vi "pulse_generator_refnum_2.vi"(1 "Stop! Refnum":refnum<vi>) -> ()   [LabVIEW 2017]
uses:
  pulse_generator_controls_refnums.ctl
  <vilib>/Utility/error.llb/DialogType.ctl
  <vilib>/DAQmx/write.llb/DAQmx Write (Digital Bool 1Line 1Point).vi
  <vilib>/DAQmx/create/channels.llb/DAQmx Create Channel (DO-Digital Output).vi
  <vilib>/DAQmx/miscellaneous.llb/DAQmx Fill In Error Info.vi
  <vilib>/DAQmx/create/channels.llb/DAQmx Create Channel (CO-Pulse Generation-Frequency).vi
  <vilib>/DAQmx/configure/timing.llb/DAQmx Timing (Implicit).vi
panel:
  in  "Pulse Generator Control Refnums":T1
  out "Stopped!":bool caption="OK"
  in  "Stop! Local":bool
  out "message":string=" INSTRUCTIONS:\r\rNormal Use:  When using subVIs that incorporate the error in/error out (or error I/O) structure, place this handler where you want to inform the user of an error, typically at the end of the I/O data path, as the last action of the program.  If the error in error? is ERROR, the handler creates a message describing the error and its source.  If the type of dialog = 1 (default), the message is displayed to the user, who can only acknowedge it.  If the type = 2, the user can acknowledge the message or abort execution; aborting a program with active I/O is not recommended.  If the type = 0, no message is displayed; this is used to process the error programmatically, and the error out cluster elements are wired to individual terminals for that reason.  \r\rOther Use:\n\r\nlocal testing.  To test the error code of a subVI or function that does not have the error I/O structure, you can wire its error code and a source string to the local error code and error source inputs.  If error in error? indicates no error and error code is not equal to 0, the local code and source are substituted for the error in values, and error? is set TRUE (ERROR)."
  in  "SwitchHelper":bool
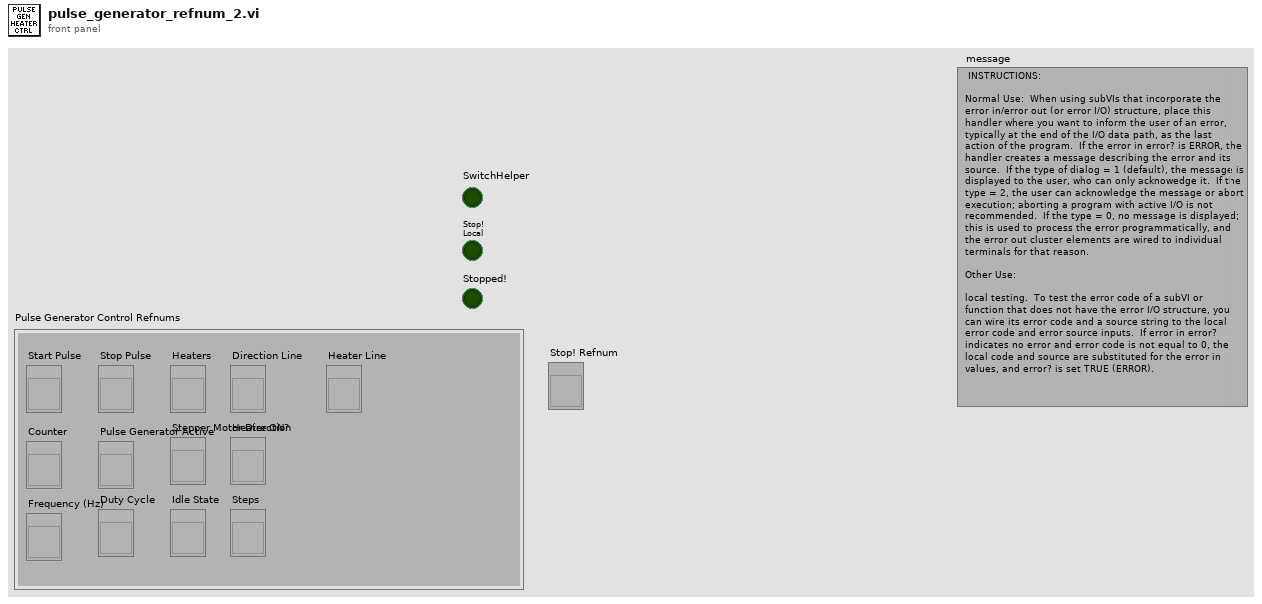
[diagram p1: front panel]
types:
  T1 = typedef "pulse_generator_controls_refnums.ctl" = cluster{"Start Pulse":refnum<vi>, "Stop Pulse":refnum<vi>, "Heaters":refnum<vi>, "Counter":refnum<vi>, "Frequency (Hz)":refnum<vi>, "Duty Cycle":refnum<vi>, "Idle State":refnum<vi>, "Pulse Generator Active":refnum<vi>, "Stepper Motor Direction":refnum<vi>, "Steps":refnum<vi>, "Direction Line":refnum<vi>, "Heater Line":refnum<vi>, "Heater ON?":refnum<vi>}
  T2 = enum8{"Enabled", "Disabled", "Disabled and Grayed Out"}
  T3 = typedef "DialogType.ctl" = u16
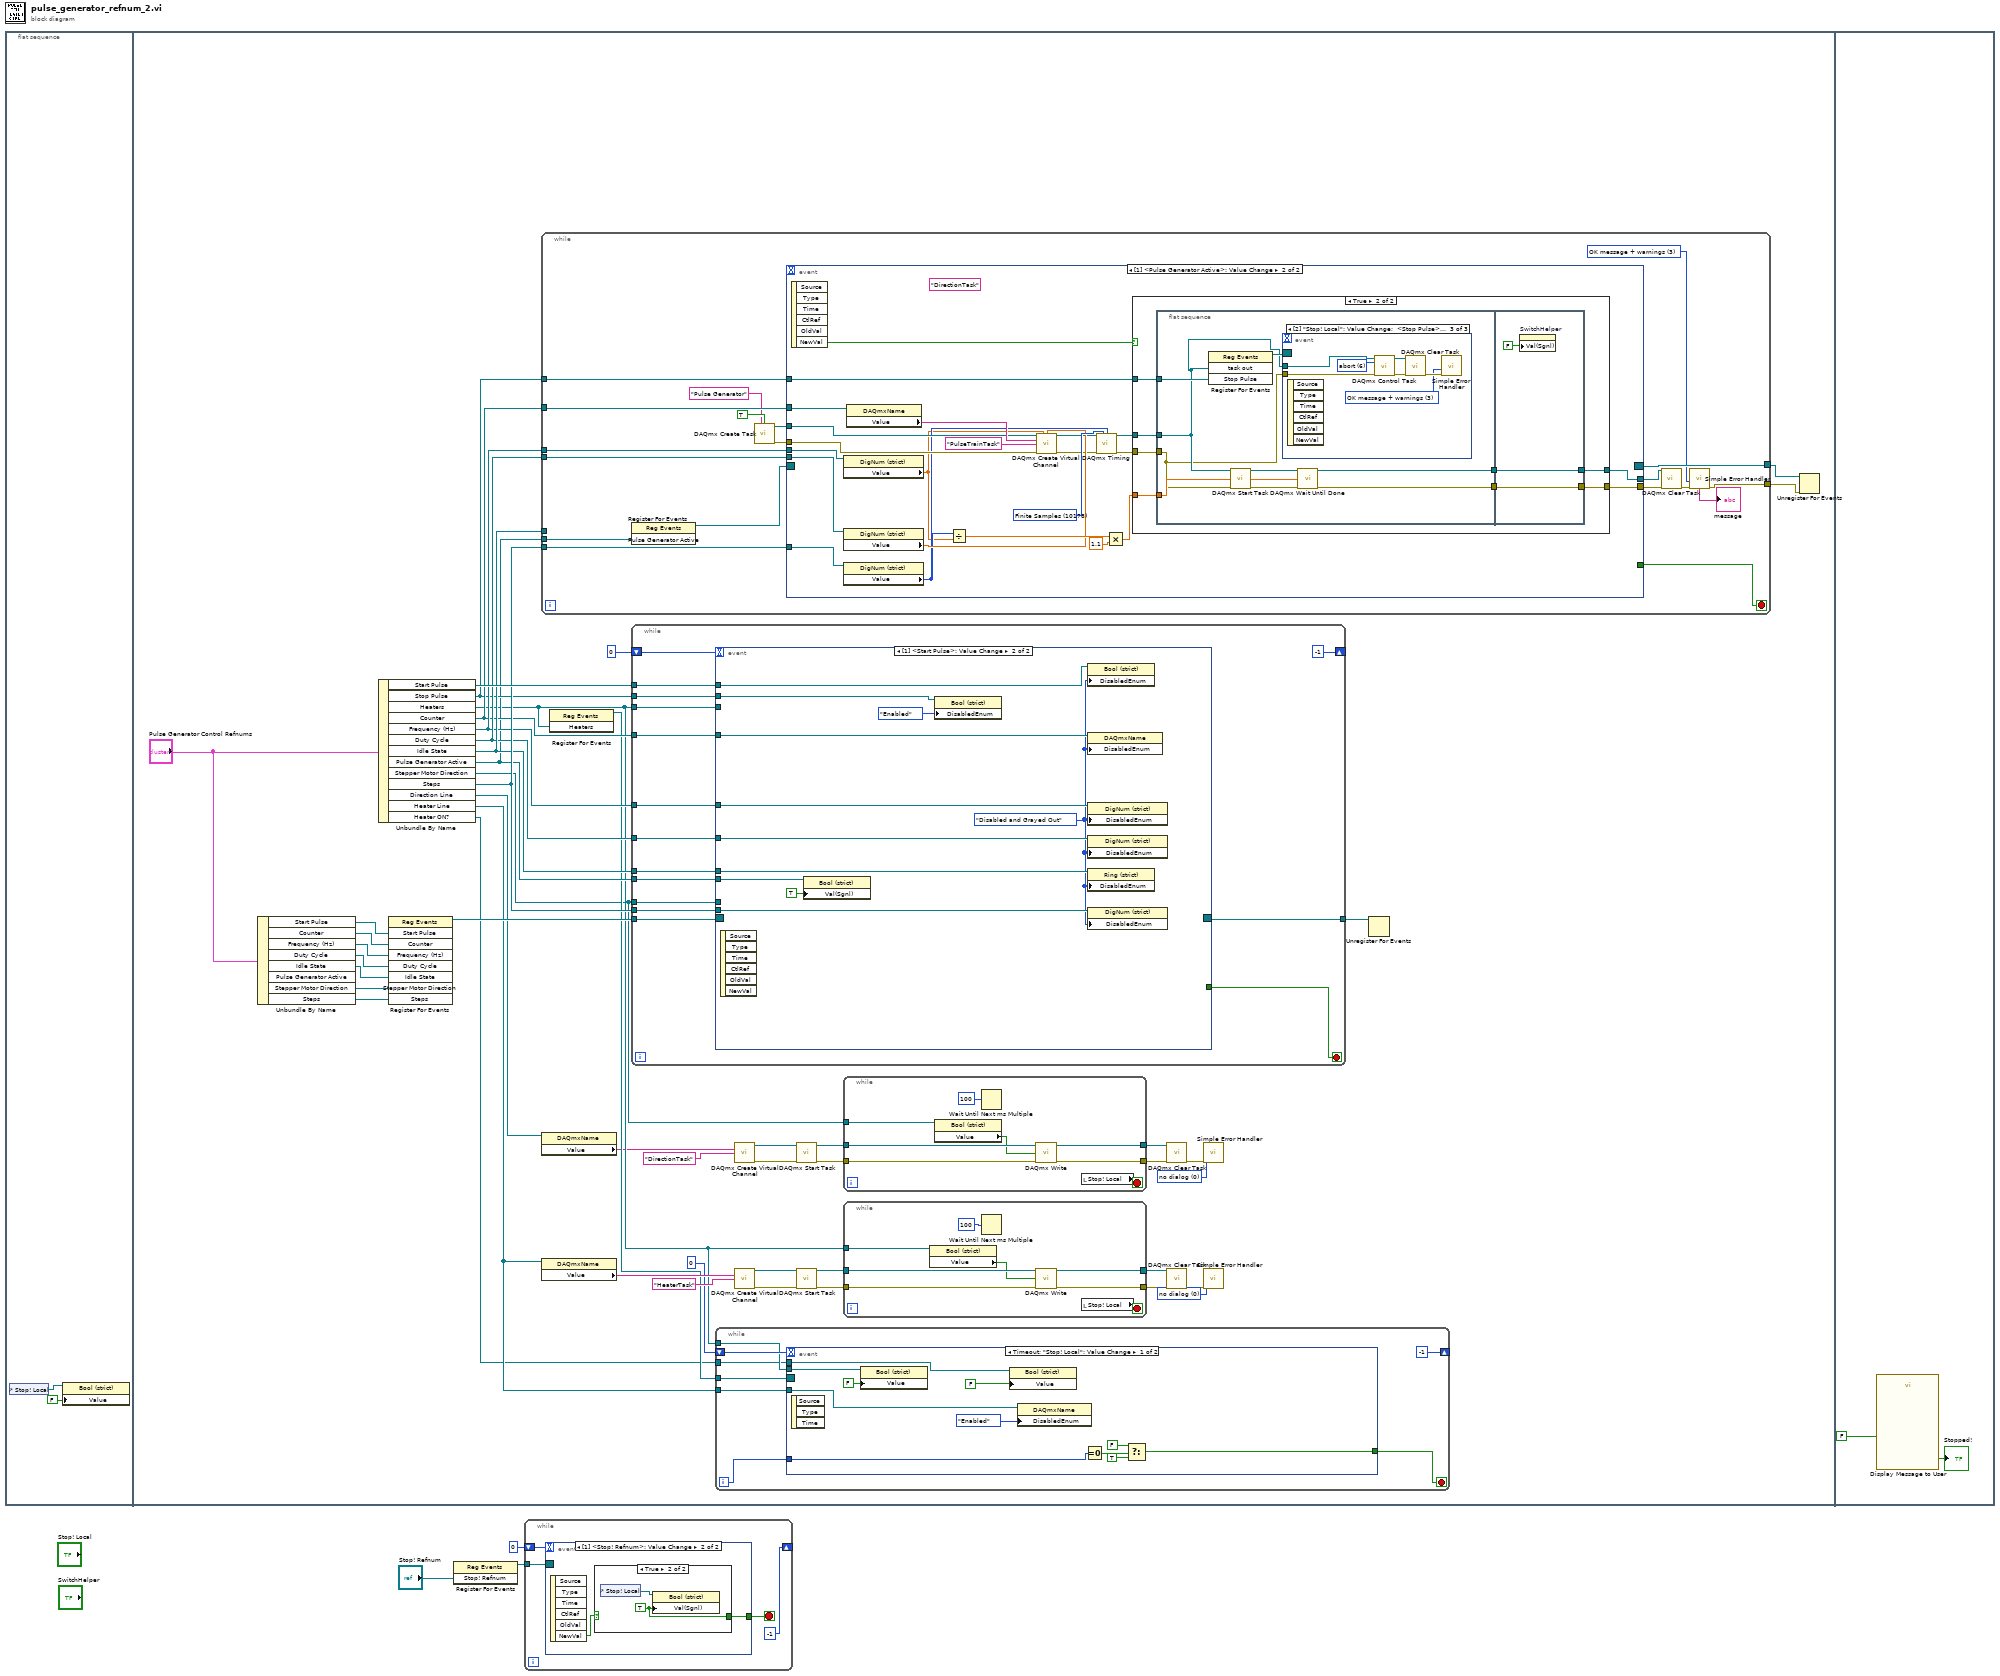
[diagram p0: block diagram]
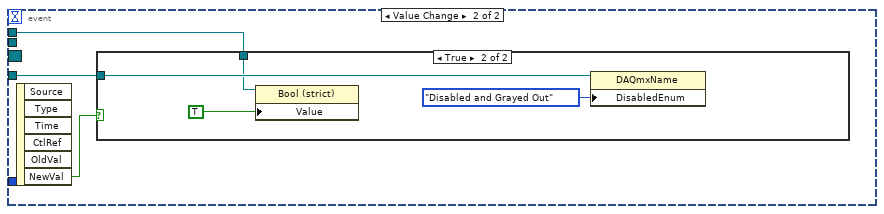
[diagram p2: hidden frame]
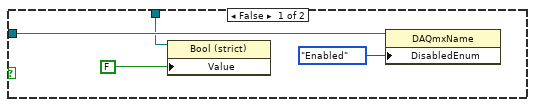
[diagram p3: hidden frame]
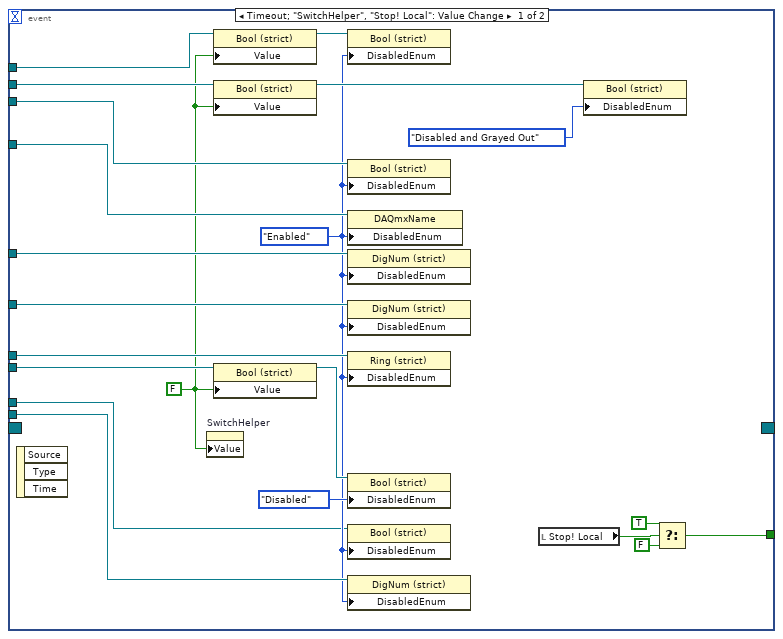
[diagram p4: hidden frame]
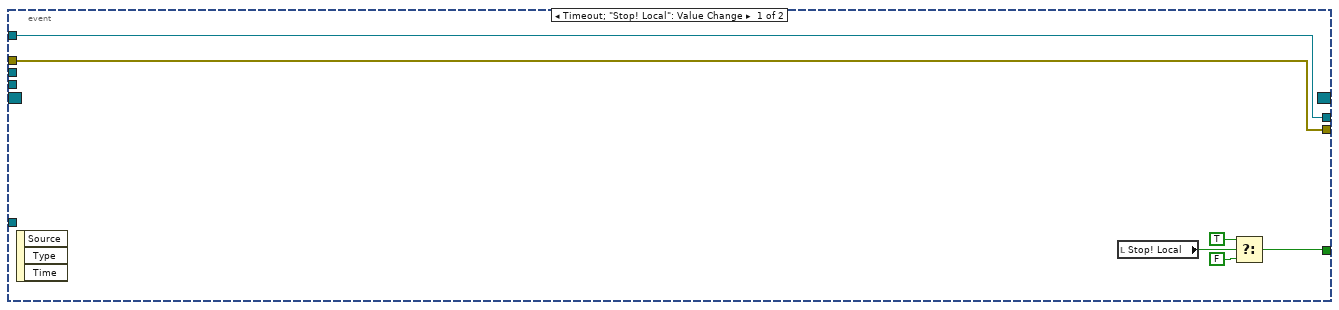
[diagram p5: hidden frame]
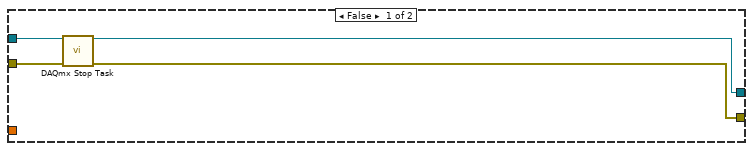
[diagram p6: hidden frame]
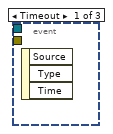
[diagram p7: hidden frame]
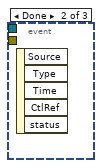
[diagram p8: hidden frame]
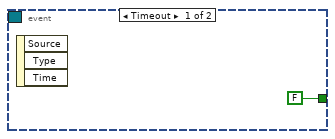
[diagram p9: hidden frame]
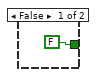
[diagram p10: hidden frame]
diagram:
  n1 = flat-sequence {
    frame #0 {
      n2 = control-ref of="Stop! Local"() -> (w4:refnum<vi>)
      n3 = property class="Bool (strict)"(reference=w4, "Value"=FALSE) -> ()  [unwired: 1 in, 2 out]
    }
    frame #1 {
      w9 = T3 0 items=["no dialog", "OK message", "continue or stop message", "OK message + warnings", "continue/stop + warnings"] ("type of dialog (OK msg:1)")
      w10 = T3 0 items=["no dialog", "OK message", "continue or stop message", "OK message + warnings", "continue/stop + warnings"] ("type of dialog (OK msg:1)")
      n4 = Unbundle By Name("Pulse Generator Control Refnums") -> ("Start Pulse"=w36:refnum<vi>, "Counter"=w51:refnum<vi>, "Frequency (Hz)"=w50:refnum<vi>, "Duty Cycle"=w49:refnum<vi>, "Idle State"=w48:refnum<vi>, "Stepper Motor Direction"=w45:refnum<vi>, "Steps"=w44:refnum<vi>)  [unwired: 1 out]
      n5 = Unbundle By Name("Pulse Generator Control Refnums") -> ("Start Pulse"=w52:refnum<vi>, "Stop Pulse"=w38:refnum<vi>, "Heaters"=w23:refnum<vi>, "Counter"=w39:refnum<vi>, "Frequency (Hz)"=w40:refnum<vi>, "Duty Cycle"=w41:refnum<vi>, "Idle State"=w42:refnum<vi>, "Pulse Generator Active"=w37:refnum<vi>, "Stepper Motor Direction"=w12:refnum<vi>, "Steps"=w43:refnum<vi>, "Direction Line"=w13:refnum<vi>, "Heater Line"=w25:refnum<vi>, "Heater ON?"=w8:refnum<vi>)
      n6 = register-events(w36, w51, w50, w49, w48, w45, w44) -> (reference out=w47:refnum<event-registration>)  [unwired: 2 in, 1 out]
      n7 = while {
        tunnel: w37 -> [w160]
        tunnel: [w162] -> w11
        tunnel: w43 -> [w155]
        tunnel: w42 -> [_]
        tunnel: w41 -> [w153]
        tunnel: w40 -> [w150]
        tunnel: w39 -> [w154]
        tunnel: w38 -> [w161]
        tunnel: [w148] -> w7
        stop <- w149 stop-if-true
        w157 = T3 3 items=["no dialog", "OK message", "continue or stop message", "OK message + warnings", "continue/stop + warnings"] ("type of dialog (OK msg:1)")
        n8 = register-events(w160) -> (reference out=w159:refnum<event-registration>)  [unwired: 2 in, 1 out]
        n9 = call <vilib>:"DAQmx Create Task.vi"("new task name"="Pulse Generator", "auto cleanup"=TRUE) -> ("task out"=w152:refnum<k21>, "error out"=w151:errorcluster)  [unwired: 12 in]
        n10 = event shown="[1] <Pulse Generator Active>: Value Change" {
          selector: w159 -> [_ _]
          dyn-events: [_ _] -> w162
          timeout: _ -> [_ _]
          tunnel: [w170 w192] -> w164
          tunnel: [w171 w193] -> w163
          tunnel: w152 -> [w171 w179]
          tunnel: w151 -> [w170 w178]
          tunnel: w161 -> [_ w191]
          tunnel: w155 -> [_ w184]
          tunnel: w154 -> [_ w182]
          tunnel: w153 -> [_ w180]
          tunnel: w150 -> [_ w172]
          tunnel: [w166 _] -> w149
          event Timeout; "Stop! Local": Value Change {
            n11 = event-data() -> ()  [unwired: 1 in, 3 out]
            n12 = local read "Stop! Local"() -> (w167:bool)
            n13 = Select(t=TRUE ("Value"), s=w167, f=FALSE ("Value")) -> (s? t:f=w166:bool)
          }
          event Value Change {
            (unwired) "DirectionTask" ("name to assign")
            w188 = 10178 items=["Finite Samples"=10178, "Continuous Samples"=10123, "Hardware Timed Single Point"=12522] ("sample mode")
            n14 = event-data() -> ("NewVal"=w194:bool)  [unwired: 1 in, 5 out]
            n15 = property class="DigNum (strict)"(reference=w172) -> ("Value"=w173:dbl)  [unwired: 1 in, 2 out]
            n16 = property class="DigNum (strict)"(reference=w180) -> ("Value"=w181:dbl)  [unwired: 1 in, 2 out]
            n17 = property class="DigNum (strict)"(reference=w184) -> ("Value"=w177:i32)  [unwired: 1 in, 2 out]
            n18 = property class="DAQmxName"(reference=w182) -> ("Value"=w183:string)  [unwired: 1 in, 2 out]
            n19 = Divide(x=w177, y=w173) -> (x/y=w186:dbl)
            n20 = call-poly <vilib>:"DAQmx Create Virtual Channel.vi"("task in"=w179, "frequency"=w173, "duty cycle"=w181, "counter"=w183, "name to assign"="PulseTrainTask", "error in"=w178) -> ("task out"=w175:refnum<k21>, "error out"=w174:errorcluster)  [unwired: 8 in]
            n21 = call-poly <vilib>:"DAQmx Timing.vi"("task/channels in"=w175, "sample mode"=w188, "samples per channel"=w177, "error in"=w174) -> ("task out"=w190:refnum<k21>, "error out"=w189:errorcluster)  [unwired: 10 in]
            n22 = Multiply(x=w186, y=1.1) -> (x*y=w185:dbl)
            n23 = case shown="True" w194 {
              tunnel: w190 -> [w198 w203]
              tunnel: w189 -> [w197 w206]
              tunnel: [w196 w205] -> w193
              tunnel: [w195 w204] -> w192
              tunnel: w191 -> [_ w200]
              tunnel: w185 -> [_ w199]
              frame False {
                n24 = call <vilib>:"DAQmx Stop Task.vi"("task/channels in"=w198, "error in"=w197) -> ("task out"=w196:refnum<k21>, "error out"=w195:errorcluster)  [unwired: 12 in]
              }
              frame True {
                n25 = flat-sequence {
                  tunnel: w206 -> [w208]
                  tunnel: w203 -> [w209]
                  tunnel: [w214] -> w202
                  tunnel: [w213] -> w201
                  tunnel: w200 -> [w211]
                  tunnel: w199 -> [w210]
                  tunnel: [w224] -> w204
                  tunnel: [w225] -> w205
                  tunnel: w202 -> [w225]
                  tunnel: w201 -> [w224]
                  frame #0 {
                    n26 = register-events(w209, w211) -> (reference out=w212:refnum<event-registration>)  [unwired: 2 in, 1 out]
                    n27 = call <vilib>:"DAQmx Start Task.vi"("task/channels in"=w209, "error in"=w208) -> ("task out"=w215:refnum<k21>, "error out"=w207:errorcluster)  [unwired: 12 in]
                    n28 = event shown="[2] \"Stop! Local\": Value Change;  <Stop Pulse>: Value Change" {
                      selector: w212 -> [_ _ _]
                      dyn-events: _ -> [_ _ _]
                      timeout: _ -> [_ _ _]
                      tunnel: w209 -> [_ _ w222]
                      tunnel: w208 -> [_ _ w221]
                      event Timeout {
                        n29 = event-data() -> ()  [unwired: 1 in, 3 out]
                      }
                      event Done {
                        n30 = event-data() -> ()  [unwired: 1 in, 5 out]
                      }
                      event "Stop! Local": Value Change {
                        w216 = T3 3 items=["no dialog", "OK message", "continue or stop message", "OK message + warnings", "continue/stop + warnings"] ("type of dialog (OK msg:1)")
                        w220 = 6 items=["verify"=2, "reserve"=4, "commit"=3, "unreserve"=5, "abort"=6] ("action")
                        n31 = event-data() -> ()  [unwired: 1 in, 6 out]
                        n32 = call <vilib>:"DAQmx Control Task.vi"("task/channels in"=w222, "action"=w220, "error in"=w221) -> ("task out"=w219:refnum<k21>, "error out"=w218:errorcluster)  [unwired: 11 in]
                        n33 = call <vilib>:"DAQmx Clear Task.vi"("task in"=w219, "error in"=w218) -> ("error out"=w217:errorcluster)  [unwired: 13 in]
                        n34 = call <vilib>:"Simple Error Handler.vi"("type of dialog (OK msg:1)"=w216, "error in (no error)"=w217) -> ()  [unwired: 3 in, 5 out]
                      }
                    }
                    n35 = call <vilib>:"DAQmx Wait Until Done.vi"("task/channels in"=w215, "timeout (sec)"=w210, "error in"=w207) -> ("task out"=w214:refnum<k21>, "error out"=w213:errorcluster)  [unwired: 11 in]
                  }
                  frame #1 {
                    n36 = property on="SwitchHelper" class="Bool (strict)"("Val(Sgnl)"=FALSE ("Value (Signaling)")) -> ()  [unwired: 2 in, 2 out]
                  }
                }
              }
            }
          }
        }
        n37 = call <vilib>:"DAQmx Clear Task.vi"("task in"=w163, "error in"=w164) -> ("error out"=w165:errorcluster)  [unwired: 13 in]
        n38 = call <vilib>:"Simple Error Handler.vi"("type of dialog (OK msg:1)"=w157, "error in (no error)"=w165) -> ("error out"=w148:errorcluster, "message"=→"message":string)  [unwired: 3 in, 3 out]
      }
      n39 = property class="DAQmxName"(reference=w13) -> ("Value"=w15:string)  [unwired: 1 in, 2 out]
      n40 = property class="DAQmxName"(reference=w25) -> ("Value"=w34:string)  [unwired: 1 in, 2 out]
      n41 = register-events(w23) -> (reference out=w26:refnum<event-registration>)  [unwired: 2 in, 1 out]
      n42 = while {
        shift-right: [-1] -> _
        shift-left: 0 -> [w114]
        tunnel: w52 -> [w112]
        tunnel: w38 -> [w111]
        tunnel: w23 -> [w101]
        tunnel: w39 -> [w107]
        tunnel: w40 -> [w106]
        tunnel: w41 -> [w105]
        tunnel: w42 -> [w104]
        tunnel: w37 -> [w110]
        tunnel: w12 -> [w103]
        tunnel: w47 -> [w109]
        tunnel: [w108] -> w46
        tunnel: w43 -> [w102]
        stop <- w100 stop-if-true
        n43 = event shown="[1] <Start Pulse>: Value Change" {
          selector: w109 -> [_ _]
          dyn-events: [_ _] -> w108
          timeout: w114 -> [_ _]
          tunnel: w112 -> [w135 w146]
          tunnel: w111 -> [w134 w140]
          tunnel: w110 -> [w133 w137]
          tunnel: w107 -> [w122 w145]
          tunnel: w106 -> [w124 w141]
          tunnel: w105 -> [w126 w144]
          tunnel: w104 -> [w127 w143]
          tunnel: w103 -> [w120 _]
          tunnel: w102 -> [w125 w142]
          tunnel: w101 -> [w123 _]
          tunnel: [w117 _] -> w100
          event Timeout; "SwitchHelper", "Stop! Local": Value Change {
            w121 = T2."Enabled" ("Disabled")
            w119 = FALSE ("Value")
            n44 = event-data() -> ()  [unwired: 1 in, 3 out]
            n45 = property on="SwitchHelper" class="Bool (strict)"("Value"=w119) -> ()  [unwired: 2 in, 2 out]
            n46 = property class="Bool (strict)"(reference=w135, "Value"=w119) -> (reference out=w132:refnum<vi>)  [unwired: 1 in, 1 out]
            n47 = property class="Bool (strict)"(reference=w134, "Value"=w119) -> (reference out=w131:refnum<vi>)  [unwired: 1 in, 1 out]
            n48 = property class="Bool (strict)"(reference=w133, "Value"=w119) -> (reference out=w130:refnum<vi>)  [unwired: 1 in, 1 out]
            n49 = property class="Bool (strict)"(reference=w132, "DisabledEnum"=w121) -> ()  [unwired: 1 in, 2 out]
            n50 = property class="Bool (strict)"(reference=w123, "DisabledEnum"=w121) -> ()  [unwired: 1 in, 2 out]
            n51 = property class="DAQmxName"(reference=w122, "DisabledEnum"=w121) -> ()  [unwired: 1 in, 2 out]
            n52 = property class="DigNum (strict)"(reference=w124, "DisabledEnum"=w121) -> ()  [unwired: 1 in, 2 out]
            n53 = property class="DigNum (strict)"(reference=w126, "DisabledEnum"=w121) -> ()  [unwired: 1 in, 2 out]
            n54 = property class="Ring (strict)"(reference=w127, "DisabledEnum"=w121) -> ()  [unwired: 1 in, 2 out]
            n55 = property class="Bool (strict)"(reference=w130, "DisabledEnum"=T2."Disabled" ("Disabled")) -> ()  [unwired: 1 in, 2 out]
            n56 = property class="Bool (strict)"(reference=w120, "DisabledEnum"=w121) -> ()  [unwired: 1 in, 2 out]
            n57 = property class="DigNum (strict)"(reference=w125, "DisabledEnum"=w121) -> ()  [unwired: 1 in, 2 out]
            n58 = local read "Stop! Local"() -> (w118:bool)
            n59 = property class="Bool (strict)"(reference=w131, "DisabledEnum"=T2."Disabled and Grayed Out" ("Disabled")) -> ()  [unwired: 1 in, 2 out]
            n60 = Select(t=TRUE ("Value"), s=w118, f=FALSE ("Value")) -> (s? t:f=w117:bool)
          }
          event Value Change {
            w139 = T2."Disabled and Grayed Out" ("Disabled")
            n61 = event-data() -> ()  [unwired: 1 in, 6 out]
            n62 = property class="Bool (strict)"(reference=w137, "Val(Sgnl)"=TRUE ("Value")) -> ()  [unwired: 1 in, 2 out]
            n63 = property class="Bool (strict)"(reference=w140, "DisabledEnum"=T2."Enabled" ("Disabled")) -> ()  [unwired: 1 in, 2 out]
            n64 = property class="Bool (strict)"(reference=w146, "DisabledEnum"=w139) -> ()  [unwired: 1 in, 2 out]
            n65 = property class="DAQmxName"(reference=w145, "DisabledEnum"=w139) -> ()  [unwired: 1 in, 2 out]
            n66 = property class="DigNum (strict)"(reference=w141, "DisabledEnum"=w139) -> ()  [unwired: 1 in, 2 out]
            n67 = property class="DigNum (strict)"(reference=w144, "DisabledEnum"=w139) -> ()  [unwired: 1 in, 2 out]
            n68 = property class="Ring (strict)"(reference=w143, "DisabledEnum"=w139) -> ()  [unwired: 1 in, 2 out]
            n69 = property class="DigNum (strict)"(reference=w142, "DisabledEnum"=w139) -> ()  [unwired: 1 in, 2 out]
          }
        }
      }
      n70 = while {
        tunnel: w26 -> [w69]
        tunnel: w25 -> [w68]
        shift-right: [-1 ("millisecond multiple")] -> _
        shift-left: 0 ("millisecond multiple") -> [w67]
        tunnel: w23 -> [w65]
        tunnel: w8 -> [w62]
        i -> [w64]
        stop <- w63 stop-if-true
        n71 = event shown="[0] Timeout;  \"Stop! Local\": Value Change" {
          selector: w69 -> [_ _]
          dyn-events: _ -> [_ _]
          timeout: w67 -> [_ _]
          tunnel: w68 -> [w79 w82]
          tunnel: w65 -> [w78 _]
          tunnel: w64 -> [w75 _]
          tunnel: [w72 _] -> w63
          tunnel: w62 -> [w70 w81]
          event Timeout; "Stop! Local": Value Change {
            n72 = event-data() -> ()  [unwired: 1 in, 3 out]
            n73 = property class="Bool (strict)"(reference=w78, "Value"=FALSE) -> ()  [unwired: 1 in, 2 out]
            n74 = property class="Bool (strict)"(reference=w70, "Value"=FALSE) -> ()  [unwired: 1 in, 2 out]
            n75 = property class="DAQmxName"(reference=w79, "DisabledEnum"=T2."Enabled" ("Disabled")) -> ()  [unwired: 1 in, 2 out]
            n76 = Equal To 0?(x=w75) -> (x = 0?=w76:bool)
            n77 = Select(t=FALSE, s=w76, f=TRUE) -> (s? t:f=w72:bool)
          }
          event Value Change {
            n78 = event-data() -> ("NewVal"=w83:bool)  [unwired: 1 in, 5 out]
            n79 = case shown="True" w83 {
              tunnel: w82 -> [w86 w90]
              tunnel: w81 -> [w85 w88]
              frame False {
                n80 = property class="Bool (strict)"(reference=w85, "Value"=FALSE) -> ()  [unwired: 1 in, 2 out]
                n81 = property class="DAQmxName"(reference=w86, "DisabledEnum"=T2."Enabled" ("Disabled")) -> ()  [unwired: 1 in, 2 out]
              }
              frame True {
                n82 = property class="Bool (strict)"(reference=w88, "Value"=TRUE) -> ()  [unwired: 1 in, 2 out]
                n83 = property class="DAQmxName"(reference=w90, "DisabledEnum"=T2."Disabled and Grayed Out" ("Disabled")) -> ()  [unwired: 1 in, 2 out]
              }
            }
          }
        }
      }
      n84 = call-poly <vilib>:"DAQmx Create Virtual Channel.vi"("lines"=w15, "name to assign"="DirectionTask") -> ("task out"=w17:refnum<k21>, "error out"=w16:errorcluster)  [unwired: 12 in]
      n85 = call-poly <vilib>:"DAQmx Create Virtual Channel.vi"("lines"=w34, "name to assign"="HeaterTask") -> ("task out"=w32:refnum<k21>, "error out"=w33:errorcluster)  [unwired: 12 in]
      n86 = call <vilib>:"DAQmx Start Task.vi"("task/channels in"=w17, "error in"=w16) -> ("task out"=w19:refnum<k21>, "error out"=w18:errorcluster)  [unwired: 12 in]
      n87 = call <vilib>:"DAQmx Start Task.vi"("task/channels in"=w32, "error in"=w33) -> ("task out"=w30:refnum<k21>, "error out"=w31:errorcluster)  [unwired: 12 in]
      n88 = while {
        tunnel: w19 -> [w61]
        tunnel: w18 -> [w60]
        tunnel: w12 -> [w58]
        tunnel: [w56] -> w20
        tunnel: [w55] -> w21
        stop <- w54 stop-if-true
        n89 = property class="Bool (strict)"(reference=w58) -> ("Value"=w57:bool)  [unwired: 1 in, 2 out]
        n90 = Wait Until Next ms Multiple(millisecond multiple=u32 100) -> ()  [unwired: 1 out]
        n91 = call-poly <vilib>:"DAQmx Write.vi"("task/channels in"=w61, "data"=w57, "error in"=w60) -> ("task out"=w56:refnum<k21>, "error out"=w55:errorcluster)  [unwired: 10 in, 1 out]
        n92 = local read "Stop! Local"() -> (w54:bool)
      }
      n93 = while {
        tunnel: w30 -> [w99]
        tunnel: w31 -> [w98]
        tunnel: w23 -> [w96]
        tunnel: [w94] -> w29
        tunnel: [w93] -> w28
        stop <- w92 stop-if-true
        n94 = property class="Bool (strict)"(reference=w96) -> ("Value"=w95:bool)  [unwired: 1 in, 2 out]
        n95 = Wait Until Next ms Multiple(millisecond multiple=u32 100) -> ()  [unwired: 1 out]
        n96 = call-poly <vilib>:"DAQmx Write.vi"("task/channels in"=w99, "data"=w95, "error in"=w98) -> ("task out"=w94:refnum<k21>, "error out"=w93:errorcluster)  [unwired: 10 in, 1 out]
        n97 = local read "Stop! Local"() -> (w92:bool)
      }
      n98 = call <vilib>:"DAQmx Clear Task.vi"("task in"=w20, "error in"=w21) -> ("error out"=w22:errorcluster)  [unwired: 13 in]
      n99 = call <vilib>:"DAQmx Clear Task.vi"("task in"=w29, "error in"=w28) -> ("error out"=w27:errorcluster)  [unwired: 13 in]
      n100 = call <vilib>:"Simple Error Handler.vi"("type of dialog (OK msg:1)"=w10, "error in (no error)"=w22) -> ()  [unwired: 3 in, 5 out]
      n101 = call <vilib>:"Simple Error Handler.vi"("type of dialog (OK msg:1)"=w9, "error in (no error)"=w27) -> ()  [unwired: 3 in, 5 out]
      n102 = Unregister For Events(event registration refnum=w46) -> ()  [unwired: 1 in, 1 out]
      n103 = Unregister For Events(event registration refnum=w11, error in=w7) -> ()  [unwired: 1 out]
    }
    frame #2 {
      n104 = call "Display Message to User"("Enable"=FALSE) -> ("OK"=→"Stopped!":bool)  [unwired: 9 in, 1 out]
    }
  }
  n105 = register-events("Stop! Refnum") -> (reference out=w2:refnum<event-registration>)  [unwired: 2 in, 1 out]
  n106 = while {
    tunnel: w2 -> [w231]
    shift-right: [-1] -> _
    shift-left: 0 -> [w230]
    stop <- w228 stop-if-true
    n107 = event shown="[1] <Stop! Refnum>: Value Change" {
      selector: w231 -> [_ _]
      dyn-events: _ -> [_ _]
      timeout: w230 -> [_ _]
      tunnel: [FALSE ("Value (Signaling)") w233] -> w228
      event Timeout {
        n108 = event-data() -> ()  [unwired: 1 in, 3 out]
      }
      event Value Change {
        n109 = event-data() -> ("NewVal"=w234:bool)  [unwired: 1 in, 5 out]
        n110 = case shown="True" w234 {
          tunnel: [FALSE ("Value (Signaling)") w237] -> w233
          frame False {
          }
          frame True {
            w237 = TRUE ("Value (Signaling)")
            n111 = control-ref of="Stop! Local"() -> (w236:refnum<vi>)
            n112 = property class="Bool (strict)"(reference=w236, "Val(Sgnl)"=w237) -> ()  [unwired: 1 in, 2 out]
          }
        }
      }
    }
  }
